vi "mWmotor_Main.vi"() -> ()   [LabVIEW 2019]
uses:
  SubVI/Automatic mode/Controller decision.ctl
  SubVI/Motor Controller/Motor Class/Motor.lvclass
  SubVI/Automation/Automation.lvclass
  SubVI/Simulation/Signaller/Signaller.lvclass
panel:
  out "Mapped Frequencuy  (GHz)":dbl format="%_6g"
  out "EIP Frequency (GHz)":dbl format="%#_7g"
  out "Current possition (rev)":dbl
  in  "Move to frequecy":bool
  in  "Set possition (rev)":dbl=0.36 min=0.0 max=4.1
  in  "Degrees":dbl=0.36 min=0.36
  in  "CCW":bool
  in  "CW":bool
  in  "stop motor":bool
  in  "Set Freq (GHz)":dbl=140.0 min=140.0 max=141.9
  out "Upper (GHz)":dbl
  out "Lower (GHz)":dbl
  in  "Range(MHz)":dbl=10.0
  in  "Center Frequency(GHz)":dbl=140.2
  in  "Seek Function":enum16{"Rate based", "Ploarization(avg) based"}(ring)
  out "Motor Action":T1
  out "Has all samples":bool
  in  "Automatic step size (rev)":dbl=0.005
  in  "Seek type":enum32{"Seek Positive", "Seek Negative"}(radio)
  in  "Start Auto control":bool
  in  "Bypass Freq check":bool
  out "Gradients":dbl[](array[numeric])
  out "Recovery sequence":string
  in  "Recovery loop stop":bool
  in  "Recovery":bool
  out "Temp alarms":bool
  in  "Start Recovery":bool
  in  "Record Data":bool
  in  "Run File name":string
  in  "Warning Sound":bool
  out "EIP Lost":string
  out "EIO Temp":string
  out "chart_temp 2":waveform(dbl)[](graph)=[{"t0"=timestamp(3772890114.31303 s since 1904-01-01), "dt"=1.0, "Y"=[0.8687935985565186]}, {"t0"=timestamp(3772890114.31303 s since 1904-01-01), "dt"=1.0, "Y"=[86.87935985565186]}, {"t0"=timestamp(3772890114.31303 s since 1904-01-01), "dt"=1.0, "Y"=[30.48853325313992]}, {"t0"=timestamp(3772890114.31303 s since 1904-01-01), "dt"=1.0, "Y"=[303.6385332531399]}] caption="EIO temperatures"
  out "T_array":dbl[](array[numeric])
  out "Polarization rate":waveform(dbl)[](graph)=[{"t0"=timestamp(3772890114.31303 s since 1904-01-01), "dt"=1.0, "Y"=[0.8687935985565186]}, {"t0"=timestamp(3772890114.31303 s since 1904-01-01), "dt"=1.0, "Y"=[86.87935985565186]}, {"t0"=timestamp(3772890114.31303 s since 1904-01-01), "dt"=1.0, "Y"=[30.48853325313992]}, {"t0"=timestamp(3772890114.31303 s since 1904-01-01), "dt"=1.0, "Y"=[303.6385332531399]}]
  out "Calibration run flag":bool
  out "New data point":bool
  out "EIPFRQ":waveform(dbl)[](graph)=[{"t0"=timestamp(3772890114.31303 s since 1904-01-01), "dt"=1.0, "Y"=[0.8687935985565186]}, {"t0"=timestamp(3772890114.31303 s since 1904-01-01), "dt"=1.0, "Y"=[86.87935985565186]}, {"t0"=timestamp(3772890114.31303 s since 1904-01-01), "dt"=1.0, "Y"=[30.48853325313992]}, {"t0"=timestamp(3772890114.31303 s since 1904-01-01), "dt"=1.0, "Y"=[303.6385332531399]}]
  out "Simulated Eventnum":i64
  out "Simulated polarization":dbl
  in  "Launch simulation":bool
  in  "Polarization data source":enum32{"NMR", "SIM"}(radio)
  out "EIO Temp reading":bool
  out "Motor alarm":bool
  out "NMR data issue":bool
  out "Loop Running":bool
  in  "NMR IP":string="192.168.24.191"
  in  "EIP":refnum<visa-resource-name>="GPIB0::5::INSTR"
  in  "ADC Port":refnum<visa-resource-name>="COM4"
  in  "stop VI":bool
  in  "Motor Port":refnum<visa-resource-name>="COM3"
  out "Current motor possition (Revolutions)":dbl(knob) caption="Current Angle" scale=0.0..4.1
  out "CCW":bool caption="CCW Limit"
  out "CW":bool caption="CW Limit"
  out "ADC Count":i32(slide) scale=0.0..32768.0
  out "ADC Count":i32
  out "Motor Running":bool
  out "Polarization":dbl
  out "Eventnum":i64
  out "Polarization Chart":waveform(dbl)[](graph)=[{"t0"=timestamp(3772890114.31303 s since 1904-01-01), "dt"=1.0, "Y"=[0.8687935985565186]}, {"t0"=timestamp(3772890114.31303 s since 1904-01-01), "dt"=1.0, "Y"=[86.87935985565186]}, {"t0"=timestamp(3772890114.31303 s since 1904-01-01), "dt"=1.0, "Y"=[30.48853325313992]}, {"t0"=timestamp(3772890114.31303 s since 1904-01-01), "dt"=1.0, "Y"=[303.6385332531399]}]
  in  "Calibration panel":bool
  in  "Calibration panel":enum32{"Page 1", "Page 2"}(tab)
  out "Lower Frequency":dbl
  out "Lower  possition":dbl
  in  "R_lower":bool
  out "New Intercept":dbl=138.611
  out "New Slope":dbl=0.864
  in  "Use_para":bool
  out "Upper  possition":dbl
  in  "cal_para":bool
  out "Upper Frequecy":dbl
  in  "R_upper":bool
  out "Intercept":dbl
  out "Slope":dbl
  in  "Set_motor":bool
  in  "File Path Control":path=path "C:/Users/ptgroup/Desktop/github/Microwave-motor-control/config.ini"
  out "Speed  (rev/s)":dbl
  in  "File Name":string
  out "Frequency (GHz)":dbl
  out "Possition (Rev)":dbl format="%_4g"
  out "New data  saved":bool
  out "Recording":bool
  in  "Stop calibration":bool
  in  "Move direction":enum32{"CCW", "CW"}(radio)
  in  "Start calibration":bool
  in  "Step size (rev)":dbl
  out "Estimated Possition":dbl
  out "error out":errorcluster
  # "Manual Motor Control"
  # "Auto control   Setup"
  # "Auto control   Parameters"
  # "Warnings"
  # "Communication  Setup"
  # "Current motor possition (Rev)"
  # "Calibration Panel"
  # "Calibration panel"
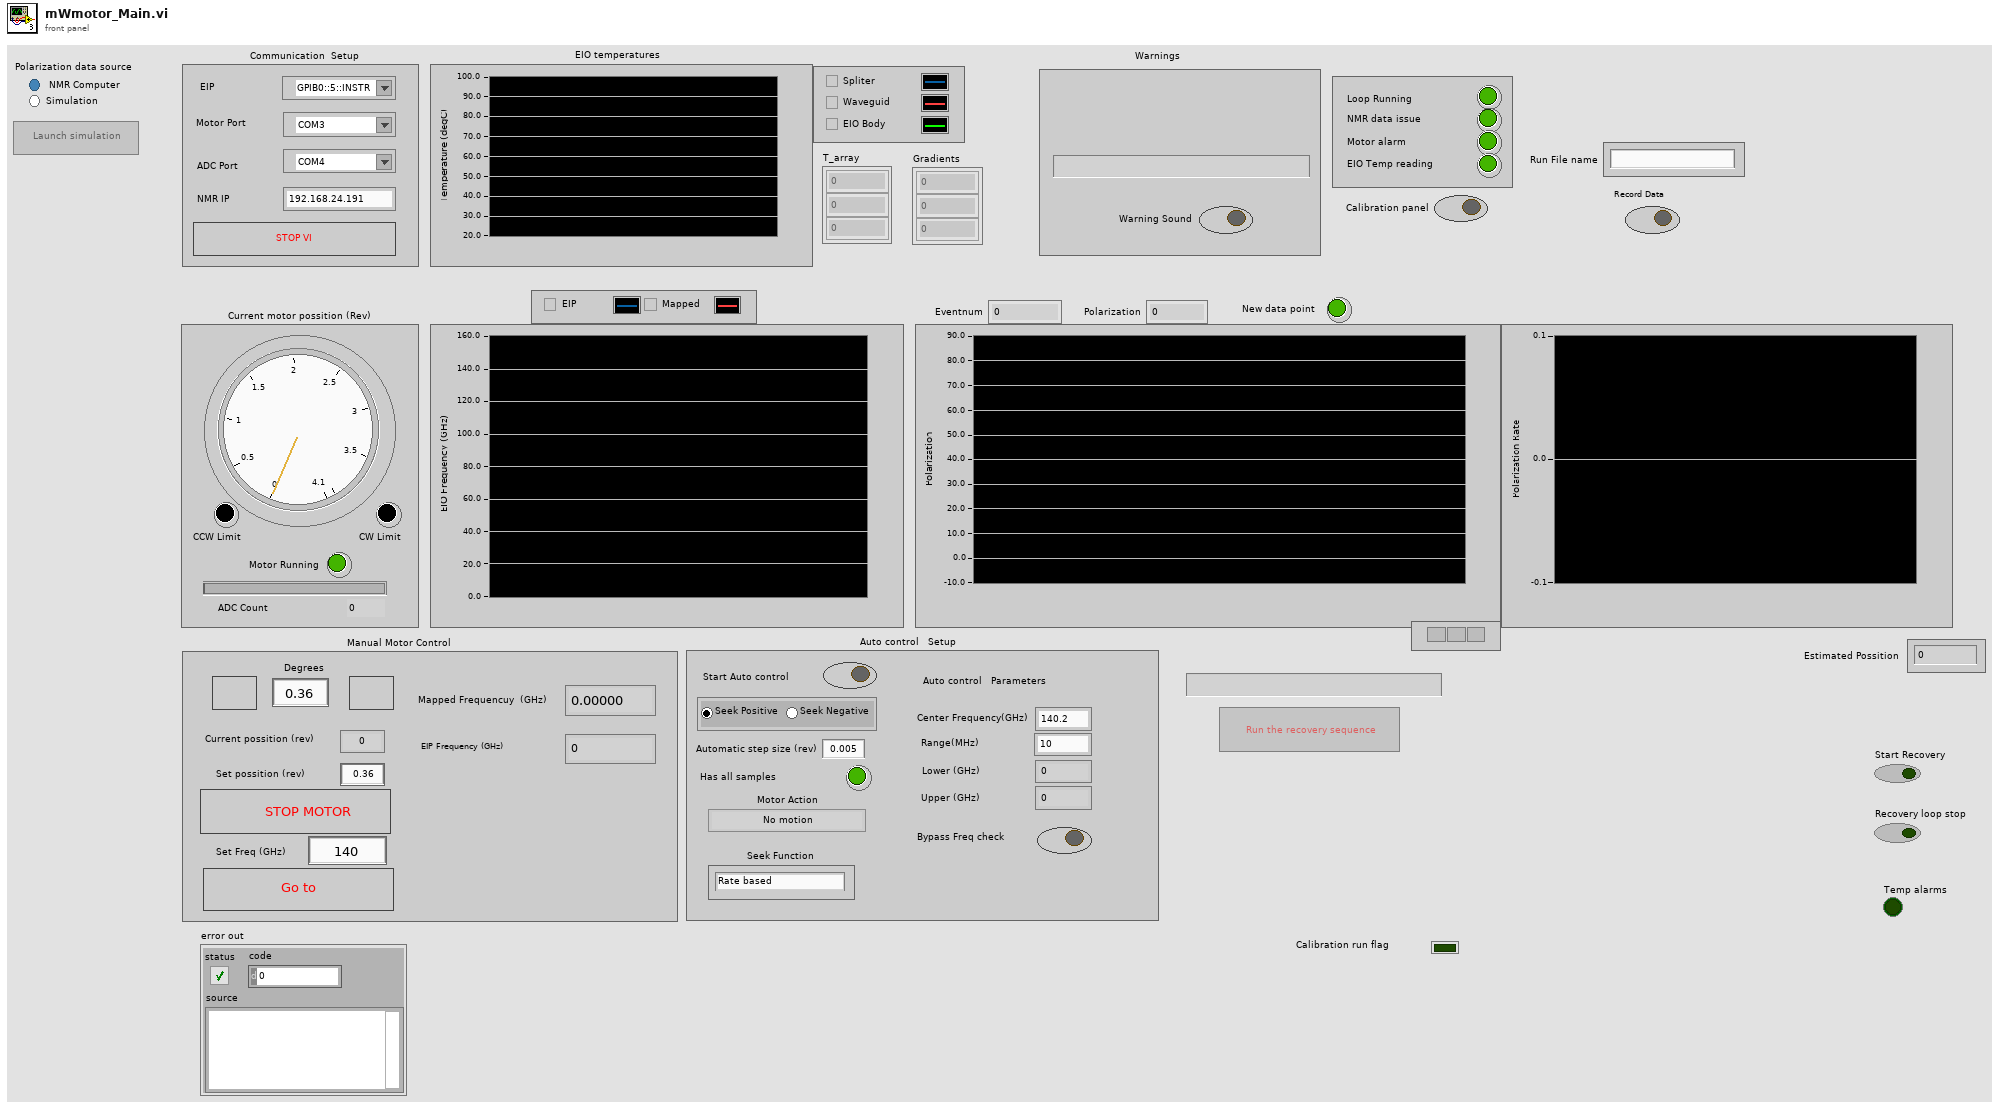
[diagram p1: front panel]
types:
  T1 = typedef "Controller decision.ctl" = enum16{"No motion", "Switch direction", "Keep current direction"}
  T2 = enum8{"Enabled", "Disabled", "Disabled and Grayed Out"}
  T3 = typedef "Sound Output Task ID.ctl" = u32
  T4 = enum32{"Bad", "Idle", "Run top level", "Running"}
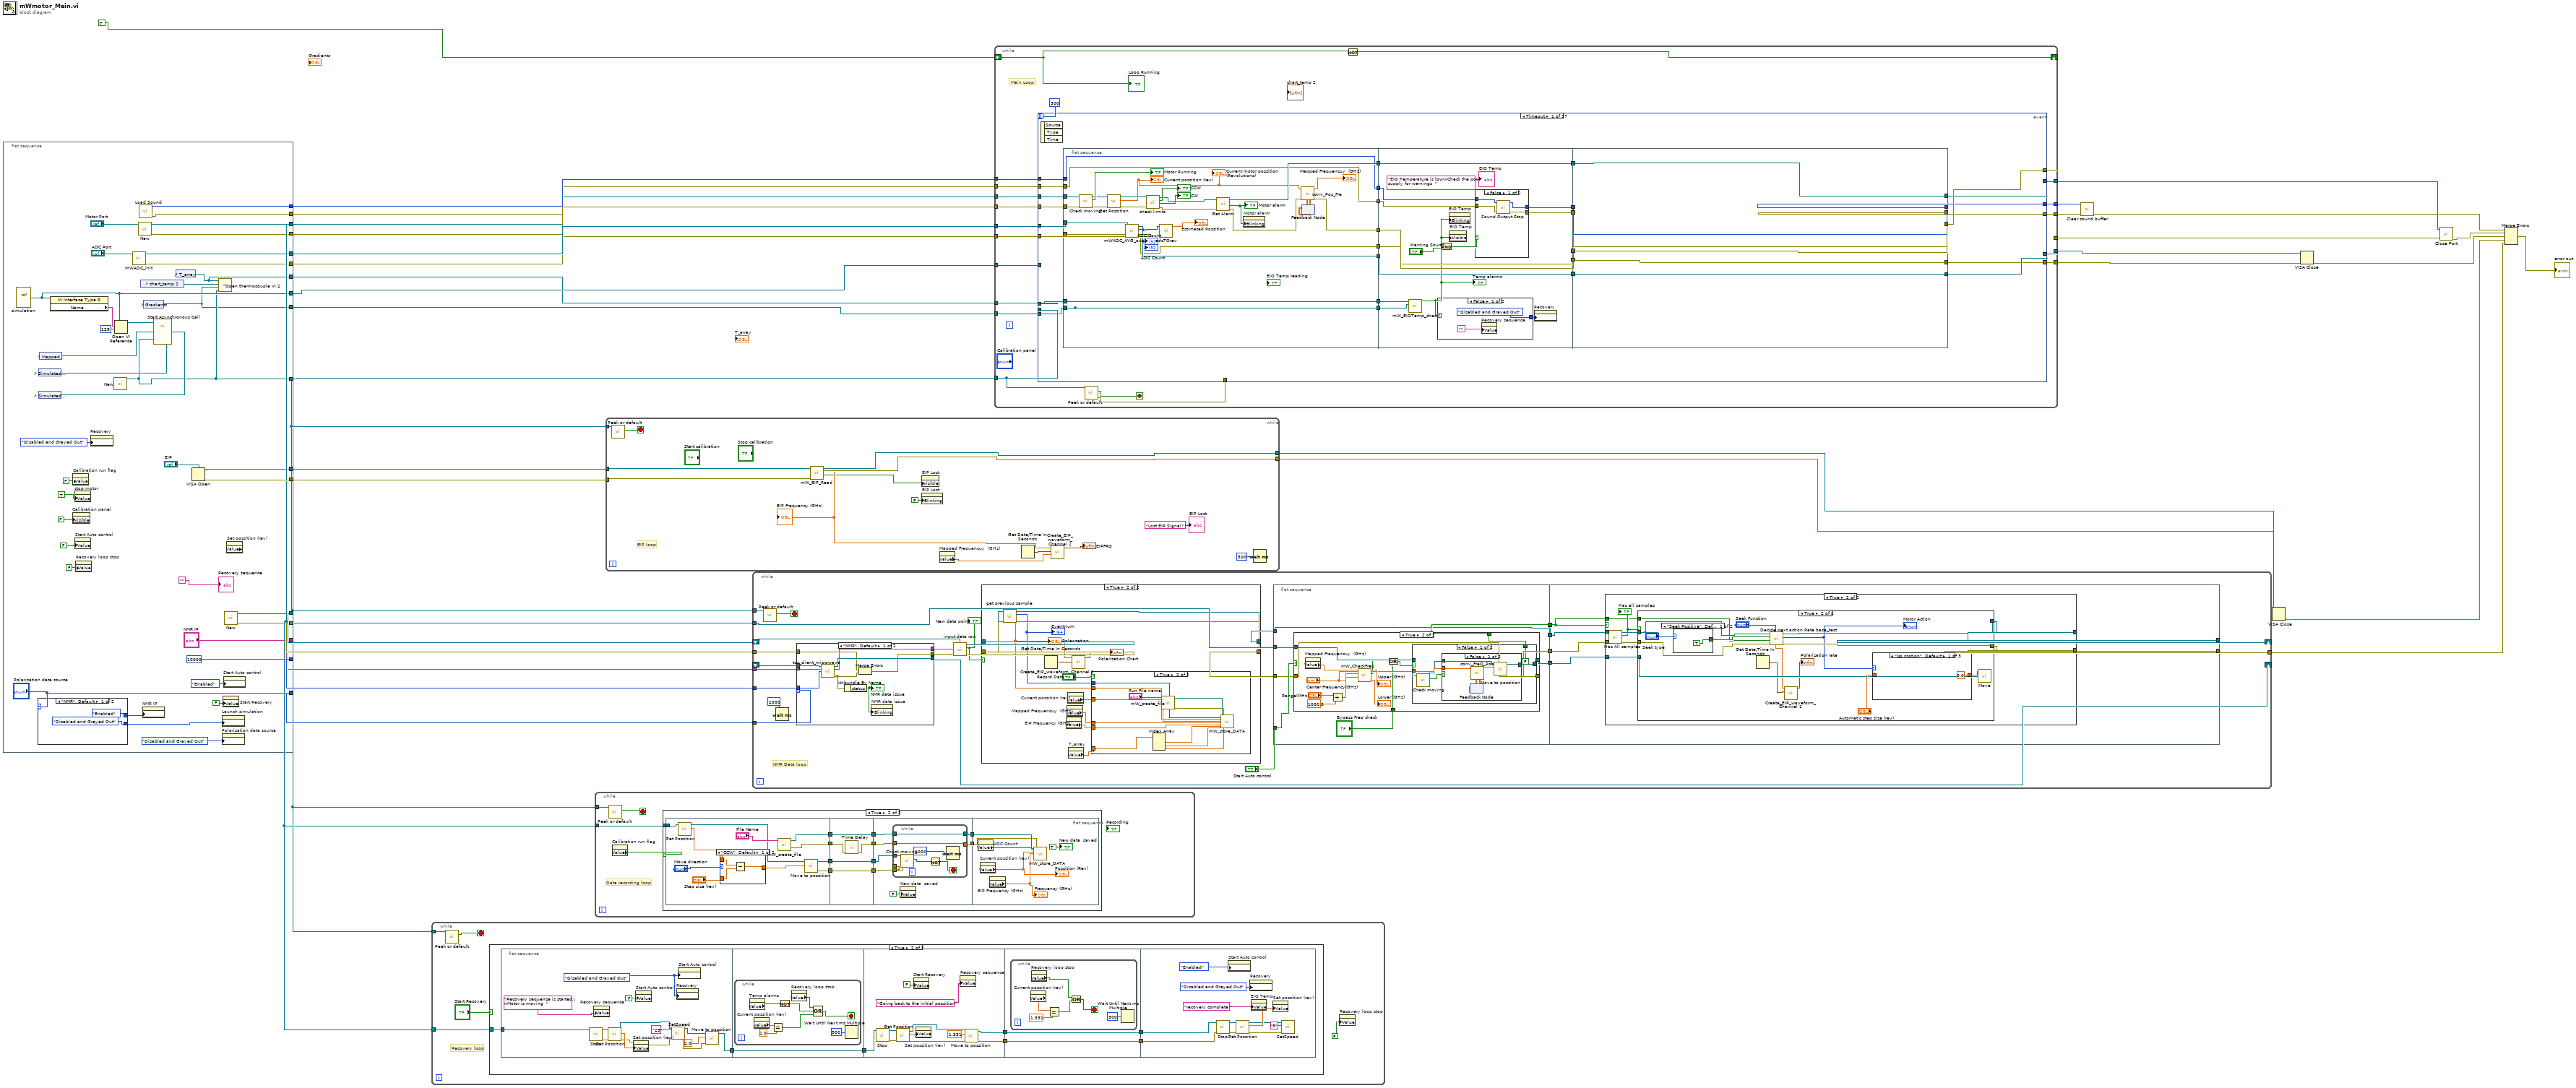
[diagram p0: block diagram]
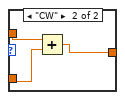
[diagram p4: hidden frame]
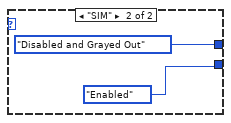
[diagram p5: hidden frame]
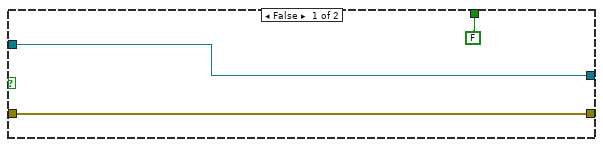
[diagram p6: hidden frame]
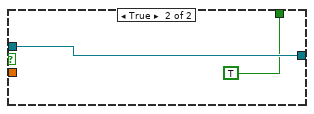
[diagram p8: hidden frame]
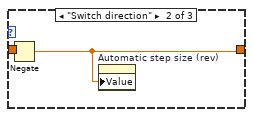
[diagram p11: hidden frame]
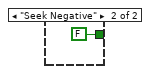
[diagram p13: hidden frame]
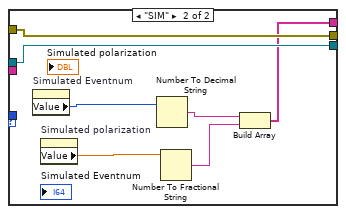
[diagram p16: hidden frame]
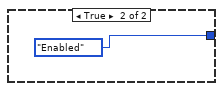
[diagram p17: hidden frame]
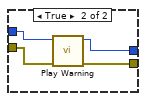
[diagram p18: hidden frame]
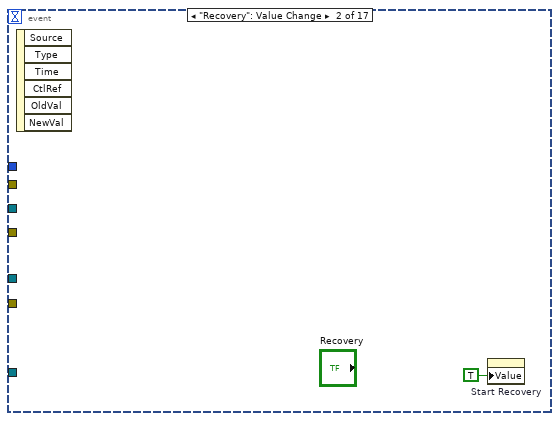
[diagram p19: hidden frame]
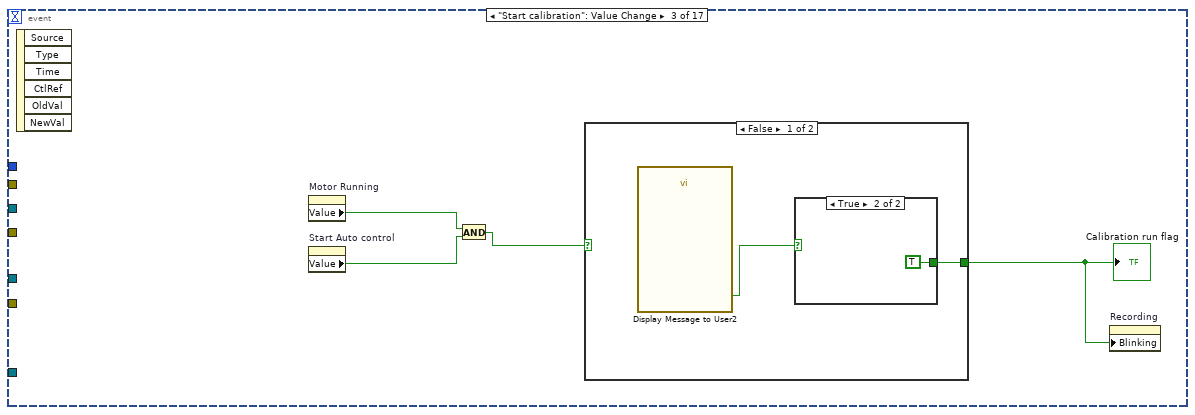
[diagram p20: hidden frame]
diagram:
  n1 = flat-sequence {
    tunnel: [w70] -> w31
    tunnel: [w69] -> w28
    tunnel: [w68] -> w25
    tunnel: [w67] -> w24
    tunnel: [w63] -> w2
    tunnel: [w62] -> w21
    tunnel: [u16 10000 ("port")] -> w16
    tunnel: [w60] -> w15
    tunnel: [w59] -> w14
    tunnel: ["NMR IP"] -> w13
    tunnel: [w55] -> w11
    tunnel: [w42] -> w3
    tunnel: ["Polarization data source"] -> w10
    tunnel: [w41] -> w9
    tunnel: [w40] -> w8
    tunnel: [w39] -> w7
    tunnel: [w33] -> w1
    frame #0 {
      n2 = vi-ref "simulation.vi"() -> (w55:refnum<vi>)
      n3 = case shown="\"NMR\", Default" "Polarization data source" {
        tunnel: [T2."Disabled and Grayed Out" ("Disabled") T2."Enabled" ("Disabled")] -> w49
        tunnel: [T2."Enabled" ("Disabled") T2."Disabled and Grayed Out" ("Disabled")] -> w47
        frame "NMR", Default {
        }
        frame "SIM" {
        }
      }
      n4 = control-ref of="Simulated Eventnum"() -> (w51:refnum<vi>)
      n5 = control-ref of="Simulated polarization"() -> (w52:refnum<vi>)
      n6 = control-ref of="Mapped Frequencuy  (GHz)"() -> (w53:refnum<vi>)
      n7 = property class="VI Interface Type 0"(reference=w55) -> ("Name"=w57:string)  [unwired: 1 in, 2 out]
      n8 = property on="Calibration panel" class="TabCtl (strict)"("Visible"=FALSE) -> ()  [unwired: 2 in, 2 out]
      n9 = property on="Calibration run flag" class="Bool (strict)"("Value"=FALSE ("Calibration run flag")) -> ()  [unwired: 2 in, 2 out]
      n10 = property on="stop motor" class="Bool (strict)"("Value"=TRUE ("Value (Signaling)")) -> ()  [unwired: 2 in, 2 out]
      n11 = property on="Start Auto control" class="Bool (strict)"("Value"=FALSE ("Start Auto control")) -> ()  [unwired: 2 in, 2 out]
      n12 = property on="Recovery loop stop" class="Bool (strict)"("Value"=FALSE ("Recovery loop stop")) -> ()  [unwired: 2 in, 2 out]
      n13 = property on="Recovery" class="Bool (strict)"("DisabledEnum"=T2."Disabled and Grayed Out" ("Disabled")) -> ()  [unwired: 2 in, 2 out]
      n14 = call "New.vi"() -> ("Signaller out"=w42:refnum<class "Signaller.lvclass">)  [unwired: 11 in]
      n15 = Open VI Reference(type specifier VI Refnum (for type only)=w55, vi path=w57, options=128) -> (vi reference=w54:refnum<vi>)  [unwired: 3 in, 1 out]
      n16 = call "mWADC_init.vi"("mWADC_Port"="ADC Port") -> ("error out"=w69:errorcluster, "reference out"=w70:refnum<visa-resource-name>)  [unwired: 9 in]
      n17 = call "New.vi"("VISA resource name"="Motor Port") -> ("error out"=w62:errorcluster, "Motor out"=w63:refnum<class "Motor.lvclass">)  [unwired: 9 in]
      n18 = call "Load Sound.vi"() -> ("error out"=w39:errorcluster, "task ID out"=w40:T3)  [unwired: 10 in]
      n19 = control-ref of="chart_temp 2"() -> (w43:refnum<vi>)
      n20 = property on="NMR IP" class="Str"("DisabledEnum"=w47) -> ()  [unwired: 2 in, 2 out]
      n21 = control-ref of="Gradients"() -> (w33:refnum<vi>)
      n22 = call-by-ref "Start Asynchronous Call"(reference=w54, "Eventnum refnum"=w51, "Polarization refnum"=w52, "Stop signaller"=w42, "Frequency refnum"=w53) -> ()  [unwired: 1 in, 2 out]
      n23 = control-ref of="T_array"() -> (w41:refnum<vi>)
      n24 = VISA Open(VISA resource name="EIP") -> (VISA resource name=w67:refnum<visa-resource-name>, error out=w68:errorcluster)  [unwired: 4 in]
      n25 = call "Open thermocouple VI 2.vi"("Signaller in"=w42, "Gradients"=w33, "chart_temp ref"=w43, "Temperaturs"=w41) -> ()  [unwired: 8 in]
      n26 = property on="Launch simulation" class="Bool"("DisabledEnum"=w49) -> ()  [unwired: 2 in, 2 out]
      n27 = property on="Polarization data source" class="RadioBtnsControl (strict)"("DisabledEnum"=T2."Disabled and Grayed Out" ("Disabled")) -> ()  [unwired: 2 in, 2 out]
      n28 = property on="Start Recovery" class="Bool (strict)"("Value"=FALSE ("Start Recovery")) -> ()  [unwired: 2 in, 2 out]
      n29 = property on="Start Auto control" class="Bool (strict)"("DisabledEnum"=T2."Enabled" ("Disabled")) -> ()  [unwired: 2 in, 2 out]
      n30 = call "New.vi"() -> ("error out"=w59:errorcluster, "Automation out"=w60:refnum<class "Automation.lvclass">)  [unwired: 10 in]
      n31 = property on="Set possition (rev)" class="DigNum (strict)" props=["Value"]() -> ()  [unwired: 2 in, 3 out]
      "Recovery sequence" <- ""
    }
  }
  n32 = while {
    tunnel: w3 -> [w79]
    tunnel: w2 -> [w77]
    stop <- w80 stop-if-true
    # "Recovery loop"
    n33 = call "Peek or default.vi"("Signaller in"=w79) -> ("Has signal?"=w80:bool)  [unwired: 8 in, 2 out]
    n34 = case shown="True" "Start Recovery" {
      tunnel: w77 -> [_ w87]
      frame False {
      }
      frame True {
        n35 = flat-sequence {
          tunnel: w87 -> [w98]
          tunnel: [w95] -> w86
          tunnel: w86 -> [w103]
          tunnel: [w103] -> w85
          tunnel: w85 -> [w120]
          tunnel: [w114] -> w83
          tunnel: [w113] -> w81
          tunnel: [w124] -> w84
          tunnel: w83 -> [w124]
          tunnel: [w123] -> w82
          tunnel: w81 -> [w123]
          tunnel: w84 -> [w138]
          tunnel: w82 -> [w137]
          frame #0 {
            w93 = T2."Disabled and Grayed Out" ("Disabled")
            n36 = call "Stop.vi"("Motor in"=w98) -> ("error out"=w101:errorcluster, "Motor out"=w100:refnum<class "Motor.lvclass">)  [unwired: 9 in]
            n37 = property on="Recovery sequence" class="Str"("Value"="Recovery sequence is started.\nMotor is moving  " ("EIO Temp")) -> ()  [unwired: 2 in, 2 out]
            n38 = call "Get Possition.vi"("error in (no error)"=w101, "Motor in"=w100) -> ("error out"=w96:errorcluster, "Revolutions"=w99:dbl, "Motor out"=w92:refnum<class "Motor.lvclass">)  [unwired: 7 in]
            n39 = property on="Set possition (rev)" class="DigNum (strict)"(error in=w96, "Value"=w99) -> (error out=w90:errorcluster)  [unwired: 1 in, 1 out]
            n40 = property on="Start Auto control" class="Bool (strict)"("Value"=FALSE ("Start Auto control")) -> ()  [unwired: 2 in, 2 out]
            n41 = call "SetSpeed.vi"("error in (no error)"=w90, "Speed"="25", "Motor in"=w92) -> ("error out"=w89:errorcluster, "Motor out"=w91:refnum<class "Motor.lvclass">)  [unwired: 7 in]
            n42 = property on="Recovery" class="Bool (strict)"("DisabledEnum"=w93) -> ()  [unwired: 2 in, 2 out]
            n43 = property on="Start Auto control" class="Bool (strict)"("DisabledEnum"=w93) -> ()  [unwired: 2 in, 2 out]
            n44 = call "Move to possition.vi"("error in (no error)"=w89, "absolute possition(rev)"=2.0, "Motor in"=w91) -> ("Motor out"=w95:refnum<class "Motor.lvclass">)  [unwired: 7 in, 1 out]
          }
          frame #1 {
            n45 = while {
              stop <- w104 stop-if-true
              n46 = property on="Temp alarms" class="Bool (strict)"() -> ("Value"=w111:bool)  [unwired: 2 in, 2 out]
              n47 = property on="Current possition (rev)" class="DigNum (strict)"() -> ("Value"=w109:dbl)  [unwired: 2 in, 2 out]
              n48 = Equal?(x=w109, y=2.0) -> (x = y?=w107:bool)
              n49 = Not(x=w111) -> (.not. x?=w106:bool)
              n50 = property on="Recovery loop stop" class="Bool (strict)"() -> ("Value"=w105:bool)  [unwired: 2 in, 2 out]
              n51 = Compound Arithmetic op=OR(w105, w106, w107) -> (w104:bool)
              n52 = Wait Until Next ms Multiple(millisecond multiple=u32 500) -> ()  [unwired: 1 out]
            }
          }
          frame #2 {
            n53 = call "Stop.vi"("Motor in"=w120) -> ("error out"=w122:errorcluster, "Motor out"=w121:refnum<class "Motor.lvclass">)  [unwired: 9 in]
            n54 = call "Get Possition.vi"("error in (no error)"=w122, "Motor in"=w121) -> ("error out"=w116:errorcluster, "Revolutions"=w119:dbl, "Motor out"=w117:refnum<class "Motor.lvclass">)  [unwired: 7 in]
            n55 = property on="Start Recovery" class="Bool (strict)"("Value"=FALSE ("Start Recovery")) -> ()  [unwired: 2 in, 2 out]
            n56 = property on="Set possition (rev)" class="DigNum (strict)"("Value"=w119) -> ()  [unwired: 2 in, 2 out]
            n57 = property on="Recovery sequence" class="Str"("Value"="Going back to the initial possition" ("EIO Temp")) -> ()  [unwired: 2 in, 2 out]
            n58 = call "Move to possition.vi"("error in (no error)"=w116, "absolute possition(rev)"=1.331, "Motor in"=w117) -> ("error out"=w114:errorcluster, "Motor out"=w113:refnum<class "Motor.lvclass">)  [unwired: 7 in]
          }
          frame #3 {
            n59 = while {
              stop <- w127 stop-if-true
              n60 = property on="Current possition (rev)" class="DigNum (strict)"() -> ("Value"=w129:dbl)  [unwired: 2 in, 2 out]
              n61 = property on="Recovery loop stop" class="Bool (strict)"() -> ("Value"=w125:bool)  [unwired: 2 in, 2 out]
              n62 = Equal?(x=w129, y=1.331) -> (x = y?=w126:bool)
              n63 = Or(x=w125, y=w126) -> (x .or. y?=w127:bool)
              n64 = Wait Until Next ms Multiple(millisecond multiple=u32 500) -> ()  [unwired: 1 out]
            }
          }
          frame #4 {
            n65 = call "Stop.vi"("error in (no error)"=w138, "Motor in"=w137) -> ("error out"=w139:errorcluster, "Motor out"=w140:refnum<class "Motor.lvclass">)  [unwired: 8 in]
            n66 = property on="Start Auto control" class="Bool (strict)"("DisabledEnum"=T2."Enabled" ("Disabled")) -> ()  [unwired: 2 in, 2 out]
            n67 = call "Get Possition.vi"("error in (no error)"=w139, "Motor in"=w140) -> ("error out"=w132:errorcluster, "Revolutions"=w141:dbl, "Motor out"=w133:refnum<class "Motor.lvclass">)  [unwired: 7 in]
            n68 = property on="Recovery" class="Bool (strict)"("DisabledEnum"=T2."Disabled and Grayed Out" ("Disabled")) -> ()  [unwired: 2 in, 2 out]
            n69 = property on="EIO Temp" class="Str"("Value"="recovery complete " ("EIO Temp")) -> ()  [unwired: 2 in, 2 out]
            n70 = property on="Set possition (rev)" class="DigNum (strict)"("Value"=w141) -> ()  [unwired: 2 in, 2 out]
            n71 = call "SetSpeed.vi"("error in (no error)"=w132, "Speed"="5", "Motor in"=w133) -> ()  [unwired: 7 in, 2 out]
          }
        }
      }
    }
    n72 = property on="Recovery loop stop" class="Bool (strict)"("Value"=FALSE ("Recovery loop stop")) -> ()  [unwired: 2 in, 2 out]
  }
  n73 = while {
    tunnel: w3 -> [w144]
    tunnel: w2 -> [w142]
    stop <- w145 stop-if-true
    # "Data recording loop"
    n74 = call "Peek or default.vi"("Signaller in"=w144) -> ("Has signal?"=w145:bool)  [unwired: 8 in, 2 out]
    n75 = property on="Calibration run flag" class="Bool (strict)"() -> ("Value"=w143:bool)  [unwired: 2 in, 2 out]
    n76 = case shown="True" w143 {
      tunnel: w142 -> [_ w150]
      frame False {
      }
      frame True {
        n77 = flat-sequence {
          tunnel: [w167] -> w154
          tunnel: [w166] -> w152
          tunnel: w150 -> [w161]
          tunnel: [w158] -> w149
          tunnel: [w157] -> w146
          tunnel: w154 -> [w177]
          tunnel: [w176] -> w153
          tunnel: w152 -> [w178]
          tunnel: [w178] -> w151
          tunnel: w149 -> [w175]
          tunnel: [w175] -> w148
          tunnel: [w174] -> w147
          tunnel: w146 -> [w174]
          tunnel: [w184] -> w156
          tunnel: w153 -> [w185]
          tunnel: w151 -> [w182]
          tunnel: [w183] -> w155
          tunnel: w148 -> [w180]
          tunnel: w147 -> [w181]
          tunnel: w156 -> [w193]
          tunnel: w155 -> [w197]
          frame #0 {
            n78 = call "Get Possition.vi"("Motor in"=w161) -> ("Revolutions"=w162:dbl, "Motor out"=w159:refnum<class "Motor.lvclass">)  [unwired: 8 in, 1 out]
            n79 = case shown="\"CCW\", Default" "Move direction" {
              tunnel: [w168 w173] -> w160
              tunnel: "Step size (rev)" -> [w169 w172]
              tunnel: w162 -> [w170 w171]
              frame "CCW", Default {
                n80 = Subtract(x=w170, y=w169) -> (x-y=w168:dbl)
              }
              frame "CW" {
                n81 = Add(x=w171, y=w172) -> (x+y=w173:dbl)
              }
            }
            n82 = call "mW_create_file.vi"("File Name"="File Name") -> ("error out"=w167:errorcluster, "dup path"=w166:path)  [unwired: 9 in]
            n83 = call "Move to possition.vi"("absolute possition(rev)"=w160, "Motor in"=w159) -> ("error out"=w158:errorcluster, "Motor out"=w157:refnum<class "Motor.lvclass">)  [unwired: 8 in]
          }
          frame #1 {
            n84 = call "Time Delay"("error in (no error)"=w177) -> ("error out"=w176:errorcluster)  [unwired: 10 in]
          }
          frame #2 {
            n85 = while {
              tunnel: [w191] -> w184
              tunnel: w185 -> [w191]
              tunnel: [w190] -> w183
              tunnel: w182 -> [w190]
              tunnel: w181 -> [w188]
              tunnel: w180 -> [w186]
              tunnel: [w186] -> _
              stop <- w192 stop-if-true
              n86 = call "Check moving.vi"("error in (no error)"=w186, "Motor in"=w188) -> ("IS Move"=w189:bool)  [unwired: 7 in, 2 out]
              n87 = Not(x=w189) -> (.not. x?=w192:bool)
              n88 = Wait (ms)(milliseconds to wait=u32 1000) -> ()  [unwired: 1 out]
            }
            n89 = property on="New data  saved" class="Bool (strict)"("Value"=FALSE ("New data  saved")) -> ()  [unwired: 2 in, 2 out]
          }
          frame #3 {
            n90 = property on="ADC Count" class="DigNum (strict)"() -> ("Value"=w196:i32)  [unwired: 2 in, 2 out]
            n91 = property on="Current possition (rev)" class="DigNum (strict)"() -> ("Value"=w195:dbl)  [unwired: 2 in, 2 out]
            "Possition (Rev)" <- w195
            n92 = property on="EIP Frequency (GHz)" class="DigNum (strict)"() -> ("Value"=w194:dbl)  [unwired: 2 in, 2 out]
            "Frequency (GHz)" <- w194
            n93 = call "mW_store_DATA.vi"("file path (dialog if empty)"=w197, "col1"=w196, "col2"=w195, "col3"=w194, "error in (no error)"=w193) -> ()  [unwired: 22 in, 1 out]
            "New data  saved" <- TRUE ("New data  saved")
          }
        }
      }
    }
  }
  n94 = while {
    tunnel: w24 -> [w209]
    tunnel: [w208] -> w27
    tunnel: [w211] -> w26
    tunnel: w25 -> [w210]
    tunnel: w3 -> [w202]
    stop <- w203 stop-if-true
    # "EIP loop"
    n95 = call "Peek or default.vi"("Signaller in"=w202) -> ("Has signal?"=w203:bool)  [unwired: 8 in, 2 out]
    n96 = call "mW_EIP_Read.vi"("error in (no error)"=w210, "VISA Refnum in"=w209) -> ("error out"=w211:errorcluster, "No Reading"=w201:bool, "Frequency"=w206:dbl, "VISA resource name out"=w208:refnum<visa-resource-name>)  [unwired: 5 in]
    "EIP Frequency (GHz)" <- w206
    n97 = property on="EIP Lost" class="Str"("Visible"=w201) -> ()  [unwired: 2 in, 2 out]
    n98 = property on="EIP Lost" class="Str"("Blinking"=FALSE) -> ()  [unwired: 2 in, 2 out]
    n99 = property on="Mapped Frequencuy  (GHz)" class="DigNum (strict)"() -> ("Value"=w199:dbl)  [unwired: 2 in, 2 out]
    n100 = Get Date/Time In Seconds() -> (seconds since 1Jan1904=w207:timestamp)
    n101 = call "Create_EIP_waveform_Channel 2.vi"("Mapped"=w199, "time"=w207, "EIP"=w206) -> ("waveform_array"=→"EIPFRQ":waveform(dbl)[])  [unwired: 8 in]
    n102 = Wait (ms)(milliseconds to wait=u32 500) -> ()  [unwired: 1 out]
    "EIP Lost" <- "Lost EIP Signal!!! " ("EIP Lost")
  }
  n103 = while {
    tunnel: w13 -> [w237]
    tunnel: w16 -> [w236]
    shift-right: [w234] -> _
    shift-left: _ -> [w235]
    tunnel: w14 -> [w227]
    shift-right: [w220] -> _
    shift-left: w15 -> [w231]
    tunnel: [w219] -> w12
    tunnel: w3 -> [w225]
    tunnel: w10 -> [w224]
    tunnel: w2 -> [w218]
    stop <- w226 stop-if-true
    # "NMR Data loop"
    n104 = call "Peek or default.vi"("Signaller in"=w225) -> ("Has signal?"=w226:bool)  [unwired: 8 in, 2 out]
    n105 = Wait (ms)(milliseconds to wait=u32 2000) -> ()  [unwired: 1 out]
    n106 = case shown="\"NMR\", Default" w224 {
      tunnel: w237 -> [w353 _]
      tunnel: w236 -> [w352 _]
      tunnel: w235 -> [w351 w359]
      tunnel: [w350 w359] -> w234
      tunnel: [w349 w357] -> w232
      tunnel: [w347 w360] -> w228
      tunnel: w227 -> [w346 w360]
      frame "NMR", Default {
        n107 = call "tcp_client_microwave.vi"("conn_id_in"=w351, "addr"=w353, "port"=w352) -> ("conn_id_out"=w350:refnum<k5>, "Raw data array"=w349:string[], "error out"=w348:errorcluster)  [unwired: 8 in, 2 out]
        n108 = Unbundle By Name(w348) -> ("status"=w345:bool)
        "NMR data issue" <- w345
        n109 = Merge Errors(w346, w348) -> (w347:errorcluster)
        n110 = property on="NMR data issue" class="Bool (strict)"("Blinking"=w345) -> ()  [unwired: 2 in, 2 out]
      }
      frame "SIM" {
        n111 = property on="Simulated Eventnum" class="DigNum (strict)"() -> ("Value"=w354:i64)  [unwired: 2 in, 2 out]
        n112 = property on="Simulated polarization" class="DigNum (strict)"() -> ("Value"=w358:dbl)  [unwired: 2 in, 2 out]
        n113 = Number To Decimal String(number=w354) -> (decimal integer string=w355:string)  [unwired: 1 in]
        n114 = Number To Fractional String(number=w358) -> (F-format string=w356:string)  [unwired: 3 in]
        n115 = Build Array(w355, w356) -> (w357:string[])
      }
    }
    n116 = call "input data row.vi"("error in (no error)"=w228, "Last row of data file"=w232, "Automation in"=w231) -> ("error out"=w230:errorcluster, "Added new data point?"=w213:bool, "Automation out"=w229:refnum<class "Automation.lvclass">)  [unwired: 4 in, 2 out]
    "New data point" <- w213
    n117 = case shown="True" w213 {
      tunnel: w230 -> [w318 w332]
      tunnel: w229 -> [w319 w331]
      tunnel: [w318 w330] -> w215
      tunnel: [w319 w329] -> w216
      frame False {
      }
      frame True {
        n118 = call "get previous sample.vi"("error in (no error)"=w332, "Automation in"=w331) -> ("error out"=w330:errorcluster, "Polarization"=w323:dbl, "Eventnum"=w324:i64, "Automation out"=w329:refnum<class "Automation.lvclass">)  [unwired: 6 in]
        "Eventnum" <- w324
        "Polarization" <- w323
        n119 = Get Date/Time In Seconds() -> (seconds since 1Jan1904=w327:timestamp)
        n120 = property on="EIP Frequency (GHz)" class="DigNum (strict)"() -> ("Value"=w320:dbl)  [unwired: 2 in, 2 out]
        n121 = property on="Mapped Frequencuy  (GHz)" class="DigNum (strict)"() -> ("Value"=w321:dbl)  [unwired: 2 in, 2 out]
        n122 = property on="Current possition (rev)" class="DigNum (strict)"() -> ("Value"=w322:dbl)  [unwired: 2 in, 2 out]
        n123 = property on="T_array" class="Arr (strict)"() -> ("Value"=w326:dbl[])  [unwired: 2 in, 2 out]
        n124 = call "Create_EIP_waveform_Channel 1.vi"("time"=w327, "Channel 1"=w323) -> ("waveform_array"=→"Polarization Chart":waveform(dbl)[])  [unwired: 9 in]
        n125 = case shown="True" "Record Data" {
          tunnel: w326 -> [_ w343]
          tunnel: w324 -> [_ w340]
          tunnel: w323 -> [_ w339]
          tunnel: w322 -> [_ w338]
          tunnel: w321 -> [_ w337]
          tunnel: w320 -> [_ w336]
          frame False {
          }
          frame True {
            n126 = Index Array(array=w343) -> (element #1=w335:dbl, element #2=w334:dbl, element #3=w333:dbl)  [unwired: 3 in]
            n127 = call "mW_create_file.vi"("File Name"="Run File name") -> ("error out"=w341:errorcluster, "dup path"=w342:path)  [unwired: 9 in]
            n128 = call "mW_store_DATA.vi"("file path (dialog if empty)"=w342, "col1"=w340, "col2"=w339, "col3"=w338, "col4"=w337, "col5"=w336, "col6"=w335, "col7"=w334, "error in (no error)"=w341, "col8"=w333) -> ()  [unwired: 17 in, 1 out]
          }
        }
      }
    }
    n129 = flat-sequence {
      tunnel: "Start Auto control" -> [w244]
      tunnel: [w245] -> w222
      tunnel: [w243] -> w221
      tunnel: w218 -> [w242]
      tunnel: [w241] -> w217
      tunnel: w216 -> [w241]
      tunnel: w215 -> [w240]
      tunnel: [w239] -> w214
      tunnel: w222 -> [w279]
      tunnel: w221 -> [w283]
      tunnel: [w282] -> w220
      tunnel: [w281] -> w219
      tunnel: w217 -> [w280]
      tunnel: w214 -> [w278]
      frame #0 {
        n130 = case shown="True" w244 {
          tunnel: w242 -> [w248 w261]
          tunnel: [w248 w262] -> w245
          tunnel: [FALSE ("Freq_in Range") w249] -> w243
          tunnel: [w246 w254] -> w239
          tunnel: w240 -> [w246 w254]
          tunnel: "Bypass Freq check" -> [_ w250]
          frame False {
          }
          frame True {
            n131 = property on="Mapped Frequencuy  (GHz)" class="DigNum (strict)"() -> ("Value"=w260:dbl)  [unwired: 2 in, 2 out]
            n132 = Divide(x="Range(MHz)", y=1000.0) -> (x/y=w259:dbl)
            n133 = call "mW_CheckFreq.vi"("Range(GHz)"=w259, "Center Frequency(GHz)"="Center Frequency(GHz)", "Current Frequency"=w260) -> ("Lower"=→"Lower (GHz)":dbl, "Freq_in Range"=w251:bool, "Upper"=→"Upper (GHz)":dbl)  [unwired: 6 in]
            n134 = Or(x=w251, y=w250) -> (x .or. y?=w252:bool)
            n135 = case shown="False" w252 {
              tunnel: [w268 w277] -> w262
              tunnel: w261 -> [w264 w277]
              tunnel: "Center Frequency(GHz)" -> [w267 _]
              tunnel: [FALSE ("Freq_in Range") TRUE ("Freq_in Range")] -> w249
              frame False {
                n136 = call "Check moving.vi"("Motor in"=w264) -> ("IS Move"=w265:bool, "Motor out"=w263:refnum<class "Motor.lvclass">)  [unwired: 8 in, 1 out]
                n137 = case shown="False" w265 {
                  tunnel: [w274 w275] -> w268
                  tunnel: w267 -> [w270 _]
                  tunnel: w263 -> [w269 w275]
                  frame False {
                    n138 = feedback #1() -> (w271:dbl[][])  [unwired: 1 in]
                    n139 = call "conv_FreQ_Pos.vi"("data_in"=w271, "Freq"=w270) -> ("Pos"=w273:dbl, "data_out"=w272:dbl[][])  [unwired: 7 in, 1 out]
                    n140 = feedback-in #1(w272) -> ()
                    n141 = call "Move to possition.vi"("absolute possition(rev)"=w273, "Motor in"=w269) -> ("Motor out"=w274:refnum<class "Motor.lvclass">)  [unwired: 8 in, 1 out]
                  }
                  frame True {
                  }
                }
              }
              frame True {
              }
            }
          }
        }
      }
      frame #1 {
        n142 = case shown="True" w283 {
          tunnel: w280 -> [w285 w294]
          tunnel: [w285 w286] -> w282
          tunnel: [w284 w287] -> w281
          tunnel: w279 -> [_ w290]
          tunnel: w283 -> [_ w289]
          tunnel: w278 -> [w284 w288]
          frame False {
          }
          frame True {
            n143 = call "Has All samples.vi"("error in (no error)"=w288, "Automation in"=w294) -> ("error out"=w293:errorcluster, "Has all samples?"=w291:bool, "Automation out"=w292:refnum<class "Automation.lvclass">)  [unwired: 7 in]
            "Has all samples" <- w291
            n144 = case shown="True" w291 {
              tunnel: w293 -> [w295 w301]
              tunnel: w292 -> [w296 w303]
              tunnel: [w296 w307] -> w286
              tunnel: [w295 w306] -> w287
              tunnel: w290 -> [_ w308]
              tunnel: w289 -> [_ w302]
              frame False {
              }
              frame True {
                n145 = case shown="\"Seek Positive\", Default" "Seek type" {
                  tunnel: [TRUE ("Seek positive polarization?") FALSE ("Seek positive polarization?")] -> w304
                  frame "Seek Positive", Default {
                  }
                  frame "Seek Negative" {
                  }
                }
                n146 = Get Date/Time In Seconds() -> (seconds since 1Jan1904=w299:timestamp)
                n147 = call "Decide next action Rate base_test.vi"("Seek Function"="Seek Function", "error in (no error)"=w301, "Seek?"=w302, "Seek positive polarization?"=w304, "Automation in"=w303) -> ("error out"=w306:errorcluster, "Decision"=w305:T1, "Automation out"=w307:refnum<class "Automation.lvclass">, "mean rate"=w297:dbl)  [unwired: 1 in, 2 out]
                "Motor Action" <- w305
                n148 = call "Create_EIP_waveform_Channel 1.vi"("time"=w299, "Channel 1"=w297) -> ("waveform_array"=→"Polarization rate":waveform(dbl)[])  [unwired: 9 in]
                n149 = case shown="\"No motion\", Default" w305 {
                  tunnel: [0.0 ("Automatic step size (rev)") w313 w315] -> w309
                  tunnel: "Automatic step size (rev)" -> [_ w314 w315]
                  frame "No motion", Default {
                  }
                  frame "Switch direction" {
                    n150 = Negate(x=w314) -> (-x=w313:dbl)
                    n151 = property on="Automatic step size (rev)" class="DigNum (strict)"("Value"=w313) -> ()  [unwired: 2 in, 2 out]
                  }
                  frame "Keep current direction" {
                  }
                }
                n152 = call "Move.vi"("degrees To move"=w309, "Motor in"=w308) -> ()  [unwired: 8 in, 2 out]
              }
            }
          }
        }
      }
    }
  }
  n153 = while {
    shift-right: [w379] -> _
    shift-left: TRUE -> [w380]
    tunnel: w31 -> [w378]
    tunnel: w28 -> [w377]
    tunnel: [w376] -> w20
    tunnel: [w375] -> w23
    tunnel: w2 -> [w374]
    tunnel: w21 -> [w373]
    tunnel: [w372] -> w18
    tunnel: [w371] -> w17
    tunnel: w11 -> [w370]
    tunnel: w3 -> [w368]
    tunnel: w9 -> [w366]
    tunnel: w8 -> [w365]
    tunnel: w7 -> [w364]
    tunnel: [w363] -> w6
    tunnel: [w362] -> w5
    tunnel: w1 -> [w361]
    stop <- w369 stop-if-true
    # "Main Loop"
    n154 = call "Peek or default.vi"("Signaller in"=w368) -> ("error out"=w367:errorcluster, "Has signal?"=w369:bool)  [unwired: 8 in, 1 out]
    n155 = event shown="[0] Timeout" {
      selector: _ -> [_ _ _ _ _ _ _ _ _ _ _ _ _ _ _ _ _]
      dyn-events: _ -> [_ _ _ _ _ _ _ _ _ _ _ _ _ _ _ _ _]
      timeout: 500 -> [_ _ _ _ _ _ _ _ _ _ _ _ _ _ _ _ _]
      tunnel: [w395 _ _ _ _ _ _ w505 w510 w523 w534 w547 _ _ w575 w585 w597] -> w376
      tunnel: [w404 _ _ _ _ _ _ _ w512 w531 _ w543 w548 w560 w582 w591 w600] -> w371
      tunnel: w378 -> [w406 _ _ _ _ _ _ _ w512 w531 _ w543 w548 w560 w582 w591 w600]
      tunnel: w377 -> [w407 _ _ _ _ _ _ w507 w513 w530 _ w542 w549 w561 w583 w590 w601]
      tunnel: [w402 _ _ _ _ _ _ w507 w513 w530 _ w542 w549 w561 w583 w590 w601] -> w375
      tunnel: w374 -> [w401 _ _ _ _ _ _ w509 w511 w529 w538 _ _ _ w581 w587 w598]
      tunnel: w373 -> [w400 _ _ _ _ _ _ w508 w510 w528 _ _ _ _ w580 w588 w599]
      tunnel: [w396 _ _ _ _ _ _ w504 w511 w521 w532 _ _ _ w573 w586 w596] -> w372
      tunnel: w370 -> [_ _ _ _ w491 _ _ _ _ _ _ _ _ _ _ _ _]
      tunnel: w368 -> [_ _ _ _ _ _ w501 _ _ _ _ _ _ _ _ _ _]
      tunnel: w367 -> [_ _ _ _ _ _ w500 _ _ _ _ _ _ _ _ _ _]
      tunnel: w366 -> [w384 _ _ _ _ _ _ _ _ _ _ _ _ _ _ _ _]
      tunnel: w365 -> [w392 _ _ _ _ _ _ _ _ _ _ _ _ _ _ _ _]
      tunnel: w364 -> [w390 _ _ _ _ _ _ _ _ _ _ _ _ _ _ _ _]
      tunnel: [w388 _ _ _ _ _ _ _ _ _ _ _ _ _ _ _ _] -> w363
      tunnel: [w386 _ _ _ _ _ _ _ _ _ _ _ _ _ _ _ _] -> w362
      tunnel: w361 -> [w382 _ _ _ _ _ _ _ _ _ _ _ _ _ _ _ _]
      event Timeout {
        n156 = event-data() -> ()  [unwired: 1 in, 3 out]
        n157 = flat-sequence {
          tunnel: w406 -> [w438]
          tunnel: [w437] -> w409
          tunnel: w407 -> [w434]
          tunnel: [w433] -> w405
          tunnel: w401 -> [w426]
          tunnel: w400 -> [w425]
          tunnel: [w418] -> w399
          tunnel: [w420] -> w394
          tunnel: [w413] -> w393
          tunnel: w392 -> [w413]
          tunnel: [w412] -> w391
          tunnel: w390 -> [w412]
          tunnel: w384 -> [w411]
          tunnel: [w411] -> w385
          tunnel: [w410] -> _
          tunnel: [w410] -> w383
          tunnel: w382 -> [w410]
          tunnel: w409 -> [w453]
          tunnel: [w453] -> w408
          tunnel: w405 -> [w452]
          tunnel: [w452] -> w403
          tunnel: w399 -> [w451]
          tunnel: [w451] -> w398
          tunnel: [w450] -> w397
          tunnel: w394 -> [w450]
          tunnel: w393 -> [w446]
          tunnel: w391 -> [w445]
          tunnel: [w444] -> w389
          tunnel: [w443] -> w387
          tunnel: w385 -> [w441]
          tunnel: w383 -> [w440]
          tunnel: [w467] -> w395
          tunnel: [w470] -> w404
          tunnel: w408 -> [w470]
          tunnel: w403 -> [w469]
          tunnel: [w469] -> w402
          tunnel: w398 -> [w467]
          tunnel: w397 -> [w468]
          tunnel: [w468] -> w396
          tunnel: [w466] -> w388
          tunnel: w389 -> [w466]
          tunnel: [w465] -> w386
          tunnel: w387 -> [w465]
          frame #0 {
            n158 = call "Check moving.vi"("error in (no error)"=w425, "Motor in"=w426) -> ("error out"=w429:errorcluster, "IS Move"=→"Motor Running":bool, "Motor out"=w424:refnum<class "Motor.lvclass">)  [unwired: 7 in]
            n159 = call "Get Possition.vi"("error in (no error)"=w429, "Motor in"=w424) -> ("error out"=w428:errorcluster, "Revolutions"=w417:dbl, "Motor out"=w423:refnum<class "Motor.lvclass">)  [unwired: 7 in]
            "Current motor possition (Revolutions)" <- w417
            "Current possition (rev)" <- w417
            n160 = call "mWADC_AVG_out.vi"("error out"=w434, "reference out"=w438) -> ("error out 2"=w433:errorcluster, "ADC_avg_out"=w435:i32, "VISA resource name out"=w437:refnum<visa-resource-name>)  [unwired: 7 in]
            "ADC Count" <- w435
            "ADC Count" <- w435
            n161 = call "check limits.vi"("error in (no error)"=w428, "Motor in"=w423) -> ("error out"=w427:errorcluster, "Negetive_L"=→"CW":bool, "Positive_L"=→"CCW":bool, "Motor out"=w422:refnum<class "Motor.lvclass">)  [unwired: 6 in]
            n162 = call "adcTOrev.vi"("ADC count"=w435) -> ("Estimated Possition"=→"Estimated Possition":dbl)  [unwired: 10 in]
            n163 = call "Get Alarm.vi"("error in (no error)"=w427, "Motor in"=w422) -> ("error out"=w419:errorcluster, "Motor alarm?"=w421:bool, "Motor out"=w420:refnum<class "Motor.lvclass">)  [unwired: 6 in, 1 out]
            "Motor alarm" <- w421
            n164 = property on="Motor alarm" class="Bool (strict)"("Blinking"=w421) -> ()  [unwired: 2 in, 2 out]
            n165 = feedback #2() -> (w415:dbl[][])  [unwired: 1 in]
            n166 = call "conv_Pos_Fre.vi"("data_in"=w415, "error in"=w419, "Pos"=w417) -> ("error out"=w418:errorcluster, "FreQ"=→"Mapped Frequencuy  (GHz)":dbl, "data_out"=w416:dbl[][])  [unwired: 6 in]
            n167 = feedback-in #2(w416) -> ()
          }
          frame #1 {
            n168 = call "mW_EIOTemp_check.vi"("Temp Gradients"=w440, "EIO temp"=w441) -> ("Temp alarms"=w442:bool)  [unwired: 9 in]
            "Temp alarms" <- w442
            n169 = case shown="False" w442 {
              tunnel: [T2."Disabled and Grayed Out" ("Disabled") T2."Enabled" ("Disabled")] -> w439
              frame False {
                n170 = property on="Recovery sequence" class="Str"("Value"="") -> ()  [unwired: 2 in, 2 out]
              }
              frame True {
              }
            }
            n171 = And(x=w442, y="Warning Sound") -> (x .and. y?=w447:bool)
            n172 = property on="EIO Temp" class="Str"("Blinking"=w442) -> ()  [unwired: 2 in, 2 out]
            n173 = property on="EIO Temp" class="Str"("Visible"=w442) -> ()  [unwired: 2 in, 2 out]
            n174 = case shown="False" w447 {
              tunnel: w446 -> [w460 w464]
              tunnel: w445 -> [w458 w463]
              tunnel: [w459 w462] -> w444
              tunnel: [w457 w461] -> w443
              frame False {
                n175 = call <vilib>:"Sound Output Stop.vi"("error in (no error)"=w458, "task ID"=w460) -> ("error out"=w457:errorcluster, "task ID out"=w459:T3)  [unwired: 8 in]
              }
              frame True {
                n176 = call "Play Warning.vi"("error in (no error)"=w463, "task ID"=w464) -> ("error out"=w461:errorcluster, "task ID 2"=w462:T3)  [unwired: 8 in]
              }
            }
            n177 = property on="Recovery" class="Bool (strict)"("DisabledEnum"=w439) -> ()  [unwired: 2 in, 2 out]
            "EIO Temp" <- "EIO Temperature is low\nCheck the power supply for warnings  " ("EIP Lost")
          }
          frame #2 {
          }
        }
      }
      event "Recovery": Value Change {
        n178 = event-data() -> ()  [unwired: 1 in, 6 out]
        n179 = property on="Start Recovery" class="Bool (strict)"("Value"=TRUE ("Start Recovery")) -> ()  [unwired: 2 in, 2 out]
      }
      event "Start calibration": Value Change {
        n180 = event-data() -> ()  [unwired: 1 in, 6 out]
        n181 = property on="Motor Running" class="Bool (strict)"() -> ("Value"=w473:bool)  [unwired: 2 in, 2 out]
        n182 = property on="Start Auto control" class="Bool (strict)"() -> ("Value"=w474:bool)  [unwired: 2 in, 2 out]
        n183 = And(x=w473, y=w474) -> (x .and. y?=w475:bool)
        n184 = case shown="False" w475 {
          tunnel: [w476 FALSE ("Calibration run flag")] -> w472
          frame False {
            n185 = call "Display Message to User2"() -> ("Yes"=w477:bool)  [unwired: 10 in, 1 out]
            n186 = case shown="True" w477 {
              tunnel: [FALSE ("Calibration run flag") TRUE ("Calibration run flag")] -> w476
              frame False {
              }
              frame True {
              }
            }
          }
          frame True {
            n187 = call "Display Message to User"() -> ()  [unwired: 10 in, 2 out]
          }
        }
        "Calibration run flag" <- w472
        n188 = property on="Recording" class="Bool (strict)"("Blinking"=w472) -> ()  [unwired: 2 in, 2 out]
      }
      event "Stop calibration": Value Change {
        n189 = event-data() -> ()  [unwired: 1 in, 6 out]
        n190 = property on="stop motor" class="Bool (strict)"("Val(Sgnl)"=FALSE ("Value (Signaling)")) -> ()  [unwired: 2 in, 2 out]
        n191 = property on="Recording" class="Bool (strict)"("Blinking"=FALSE) -> ()  [unwired: 2 in, 2 out]
        n192 = property on="Calibration run flag" class="Bool (strict)"("Value"=FALSE ("Calibration run flag")) -> ()  [unwired: 2 in, 2 out]
      }
      event "Launch simulation": Value Change {
        n193 = event-data() -> ()  [unwired: 1 in, 6 out]
        n194 = invoke class="VI (strict)" method="FP.Open"(reference=w491) -> (reference out=w485:refnum<vi>, error out=w484:errorcluster)  [unwired: 4 in, 3 out]
        n195 = property class="VI Interface Type 0"(reference=w485, error in=w484) -> (reference out=w490:refnum<vi>, error out=w489:errorcluster, "Exec.State"=w488:T4)
        n196 = Equal?(x=w488, y=T4."Idle" ("Execution:State")) -> (x = y?=w486:bool)
        n197 = case shown="True" w486 {
          tunnel: w490 -> [_ w495]
          tunnel: w489 -> [w492 w494]
          tunnel: [w492 w493] -> _
          frame False {
          }
          frame True {
            n198 = invoke class="VI (strict)" method="Run VI"(reference=w495, error in=w494, "Wait until done"=FALSE ("Wait Until Done"), "Auto Dispose Ref"=TRUE ("Auto Dispose Reference")) -> (error out=w493:errorcluster)  [unwired: 1 in, 4 out]
          }
        }
      }
      event "Calibration panel": Value Change {
        n199 = event-data() -> ()  [unwired: 1 in, 6 out]
        n200 = property on="Calibration panel" class="TabCtl (strict)"("Visible"="Calibration panel") -> ()  [unwired: 2 in, 2 out]
        n201 = call "Close thermocouple VI.vi"() -> ()  [unwired: 11 in, 1 out]
      }
      event "stop VI": Value Change {
        (unwired) TRUE ("stop")
        n202 = event-data() -> ()  [unwired: 1 in, 3 out]
        n203 = property on="Polarization data source" class="RadioBtnsControl (strict)"("DisabledEnum"=T2."Enabled" ("Disabled")) -> ()  [unwired: 2 in, 2 out]
        n204 = call "Signal.vi"("error in (no error)"=w500, "Signaller in"=w501) -> ()  [unwired: 8 in, 2 out]
      }
      event "stop motor": Value Change {
        n205 = event-data() -> ()  [unwired: 1 in, 5 out]
        n206 = call "Stop.vi"("error in (no error)"=w508, "Motor in"=w509) -> ("error out"=w506:errorcluster, "Motor out"=w504:refnum<class "Motor.lvclass">)  [unwired: 8 in]
        n207 = call "Get Possition.vi"("error in (no error)"=w506, "Motor in"=w504) -> ("error out"=w505:errorcluster, "Revolutions"=w503:dbl)  [unwired: 7 in, 1 out]
        n208 = property on="Set possition (rev)" class="DigNum (strict)"("Value"=w503) -> ()  [unwired: 2 in, 2 out]
        n209 = property on="Recovery loop stop" class="Bool (strict)"("Value"=TRUE ("Recovery loop stop")) -> ()  [unwired: 2 in, 2 out]
      }
      event "cal_para": Value Change {
        n210 = event-data() -> ()  [unwired: 1 in, 5 out]
        n211 = property on="Upper  possition" class="DigNum (strict)"() -> ("Value"=w516:dbl)  [unwired: 2 in, 2 out]
        n212 = property on="Lower  possition" class="DigNum (strict)"() -> ("Value"=w517:dbl)  [unwired: 2 in, 2 out]
        n213 = property on="Lower Frequency" class="DigNum (strict)"() -> ("Value"=w518:dbl)  [unwired: 2 in, 2 out]
        n214 = property on="Upper Frequecy" class="DigNum (strict)"() -> ("Value"=w519:dbl)  [unwired: 2 in, 2 out]
        n215 = formula code="m=(y2-y1)/(x2-x1);\nc=y2-m*x2;"("x1"=w517, "y1"=w518, "x2"=w516, "y2"=w519) -> ("m"=→"New Slope":dbl, "c"=→"New Intercept":dbl)
      }
      event "CW": Value Change {
        n216 = event-data() -> ()  [unwired: 1 in, 6 out]
        n217 = local read "Degrees"() -> (w526:dbl)
        n218 = Divide(x=w526, y=360.0) -> (x/y=w525:dbl)
        n219 = call "Move.vi"("error in (no error)"=w528, "degrees To move"=w525, "Motor in"=w529) -> ("error out"=w524:errorcluster, "Motor out"=w522:refnum<class "Motor.lvclass">)  [unwired: 7 in]
        n220 = call "Get Possition.vi"("error in (no error)"=w524, "Motor in"=w522) -> ("error out"=w523:errorcluster, "Revolutions"=w520:dbl, "Motor out"=w521:refnum<class "Motor.lvclass">)  [unwired: 7 in]
        n221 = property on="Set possition (rev)" class="DigNum (strict)"("Value"=w520) -> ()  [unwired: 2 in, 2 out]
      }
      event "Set_motor": Value Change {
        n222 = event-data() -> ()  [unwired: 1 in, 6 out]
        n223 = call "mWmotor_set_motor_para.vi"("configuration file path"="File Path Control") -> ("Intercept"=→"Intercept":dbl, "Slope"=→"Slope":dbl, "Speed"=w537:string)  [unwired: 8 in]
        n224 = call "SetSpeed.vi"("Speed"=w537, "Motor in"=w538) -> ("error out"=w535:errorcluster, "Motor out"=w536:refnum<class "Motor.lvclass">)  [unwired: 8 in]
        n225 = call "Get Speed.vi"("error in (no error)"=w535, "Motor in"=w536) -> ("error out"=w534:errorcluster, "Speed"=→"Speed  (rev/s)":dbl, "Motor out"=w532:refnum<class "Motor.lvclass">)  [unwired: 7 in]
      }
      event "Use_para": Value Change {
        n226 = event-data() -> ()  [unwired: 1 in, 6 out]
        n227 = property on="File Path Control" class="Path"() -> ("Value"=w546:path)  [unwired: 2 in, 2 out]
        n228 = property on="New Slope" class="DigNum (strict)"() -> ("Value"=w544:dbl)  [unwired: 2 in, 2 out]
        n229 = property on="New Intercept" class="DigNum (strict)"() -> ("Value"=w545:dbl)  [unwired: 2 in, 2 out]
        n230 = property on="Intercept" class="DigNum (strict)"("Value"=w545) -> ()  [unwired: 2 in, 2 out]
        n231 = property on="Slope" class="DigNum (strict)"("Value"=w544) -> ()  [unwired: 2 in, 2 out]
        n232 = call "mWmotor_write_fitparameter.vi"("Intercept"=w545, "Slope"=w544, "configuration file path"=w546) -> ("error out"=w547:errorcluster)  [unwired: 8 in]
      }
      event "R_lower": Value Change {
        w553 = 100
        n233 = event-data() -> ()  [unwired: 1 in, 6 out]
        n234 = property on="EIP Frequency (GHz)" class="DigNum (strict)"() -> ("Value"=w551:dbl)  [unwired: 2 in, 2 out]
        n235 = property on="Current possition (rev)" class="DigNum (strict)"() -> ("Value"=→"Lower  possition":dbl)  [unwired: 2 in, 2 out]
        n236 = for {
          N: w553 -> [_]
          shift-right: [w558] -> w554
          shift-left: 0.0 ("y") -> [w559]
          tunnel: w551 -> [w557]
          n237 = Add(x=w559, y=w557) -> (x+y=w558:dbl)
        }
        n238 = Divide(x=w554, y=w553) -> (x/y=→"Lower Frequency":dbl)
        n239 = Wait (ms)(milliseconds to wait=u32 100) -> ()  [unwired: 1 out]
      }
      event "R_upper": Value Change {
        w566 = 100
        n240 = event-data() -> ()  [unwired: 1 in, 6 out]
        n241 = property on="EIP Frequency (GHz)" class="DigNum (strict)"() -> ("Value"=w563:dbl)  [unwired: 2 in, 2 out]
        n242 = property on="Current possition (rev)" class="DigNum (strict)"() -> ("Value"=→"Upper  possition":dbl)  [unwired: 2 in, 2 out]
        n243 = for {
          N: w566 -> [_]
          shift-right: [w570] -> w567
          shift-left: 0.0 ("y") -> [w571]
          tunnel: w563 -> [w569]
          n244 = Add(x=w571, y=w569) -> (x+y=w570:dbl)
        }
        n245 = Divide(x=w567, y=w566) -> (x/y=→"Upper Frequecy":dbl)
        n246 = Wait (ms)(milliseconds to wait=u32 100) -> ()  [unwired: 1 out]
      }
      event "CCW": Value Change {
        n247 = event-data() -> ()  [unwired: 1 in, 3 out]
        n248 = Negate(x="Degrees") -> (-x=w578:dbl)
        n249 = Divide(x=w578, y=360.0) -> (x/y=w579:dbl)
        n250 = call "Move.vi"("error in (no error)"=w580, "degrees To move"=w579, "Motor in"=w581) -> ("error out"=w576:errorcluster, "Motor out"=w574:refnum<class "Motor.lvclass">)  [unwired: 7 in]
        n251 = call "Get Possition.vi"("error in (no error)"=w576, "Motor in"=w574) -> ("error out"=w575:errorcluster, "Revolutions"=w572:dbl, "Motor out"=w573:refnum<class "Motor.lvclass">)  [unwired: 7 in]
        n252 = property on="Set possition (rev)" class="DigNum (strict)"("Value"=w572) -> ()  [unwired: 2 in, 2 out]
      }
      event "Set possition (rev)": Value Change {
        n253 = event-data() -> ()  [unwired: 1 in, 3 out]
        n254 = call "Move to possition.vi"("error in (no error)"=w588, "absolute possition(rev)"="Set possition (rev)", "Motor in"=w587) -> ("error out"=w585:errorcluster, "Motor out"=w586:refnum<class "Motor.lvclass">)  [unwired: 7 in]
      }
      event "Move to frequecy": Value Change {
        n255 = event-data() -> ()  [unwired: 1 in, 3 out]
        n256 = feedback #3() -> (w592:dbl[][])  [unwired: 1 in]
        n257 = call "conv_FreQ_Pos.vi"("data_in"=w592, "Freq"="Set Freq (GHz)") -> ("Pos"=w595:dbl, "data_out"=w593:dbl[][])  [unwired: 7 in, 1 out]
        n258 = feedback-in #3(w593) -> ()
        n259 = call "Move to possition.vi"("error in (no error)"=w599, "absolute possition(rev)"=w595, "Motor in"=w598) -> ("error out"=w597:errorcluster, "Motor out"=w596:refnum<class "Motor.lvclass">)  [unwired: 7 in]
      }
    }
    n260 = Not(x=w380) -> (.not. x?=w379:bool)
    "Loop Running" <- w380
  }
  n261 = call "Clear sound buffer.vi"("error in (no error)"=w5, "task ID"=w6) -> ("error out"=w4:errorcluster)  [unwired: 9 in]
  n262 = VISA Close(VISA resource name=w27, error in (no error)=w26) -> (error out=w22:errorcluster)
  n263 = VISA Close(VISA resource name=w17, error in (no error)=w23) -> (error out=w30:errorcluster)
  n264 = call "Close Port.vi"("error in (no error)"=w20, "Motor in"=w18) -> ("error out"=w19:errorcluster)  [unwired: 9 in]
  n265 = Merge Errors(w4, w19, w30, w22, w12) -> (→"error out":errorcluster)
